vi "visuallyInspectPositionListResults2.vi"() -> ()   [LabVIEW 2016]
uses:
  <vilib>/Utility/file.llb/Write Delimited Spreadsheet (DBL).vi
  <vilib>/regexp/Match Regular Expression.xnode
  <vilib>/vision/driver/NI_Vision_Acquisition_Software.lvlib
panel:
  in  "Ncaptures":i32=10
  in  "Scan height?":bool=TRUE
  in  "Stepsize [um]":dbl=200.0
  in  "Focusing test range [mm]":dbl=0.8
  in  "milliseconds to wait":u32=5000
  in  "Camera gain":dbl(slide)=5.019455252918288 scale=0.0..16.0
  in  "Nloops":i32=1
  in  "Home?":bool
  in  "Path to save collected images":path=path "C:/Users/Aerotech/Documents/Stave Assembly Records/2017-03-30/ChangeHeight/images"
  out "Finished!":bool
  out "Image #":i32=319
  out "Error report":errorcluster
  out "Most recently collected image":T1(plugin-control)
  out "XYZ Stage Current Position":T2={"X [-750, 750 mm]"=122.51800503908298, "Y [-150, 30 mm]"=-145.62509155644523, "Z [-50, 50 mm]"=10.9688762056}
  in  "Axes Speeds [mm/s]":T3={"X Speed"=10.0, "Y Speed"=10.0, "Z Speed"=10.0}
  out "Moving":bool
  in  "Camera Name":refnum<k21>="cam1" caption="IMAQdx Session"
  in  "Object Location [mm]":T4={"Go to X"=122.518, "Go to Y"=-145.6251, "Go to Z"=10.9689}
  in  "error in (no error)":errorcluster
  in  "Set of Coordinates to Process":dbl[][](array[numeric])=[[122.518, -50.0451, 9.5689], [122.518, -50.0451, 9.5689], [122.518, -50.0451, 9.5689], [122.518, -50.0451, 9.5689], [122.518, -50.0451, 9.5689], [122.518, -50.0451, 9.5689], [122.518, -50.0451, 9.5689], [122.518, -50.0451, 9.5689], [122.518, -50.0451, 9.5689], [122.518, -50.0451, 9.5689], [122.518, -50.0451, 9.768899999999999], [122.518, -50.0451, 9.768899999999999], [122.518, -50.0451, 9.768899999999999], [122.518, -50.0451, 9.768899999999999], [122.518, -50.0451, 9.768899999999999], [122.518, -50.0451, 9.768899999999999], [122.518, -50.0451, 9.768899999999999], [122.518, -50.0451, 9.768899999999999], [122.518, -50.0451, 9.768899999999999], [122.518, -50.0451, 9.768899999999999], [122.518, -50.0451, 9.9689], [122.518, -50.0451, 9.9689], [122.518, -50.0451, 9.9689], [122.518, -50.0451, 9.9689], [122.518, -50.0451, 9.9689], [122.518, -50.0451, 9.9689], [122.518, -50.0451, 9.9689], [122.518, -50.0451, 9.9689], [122.518, -50.0451, 9.9689], [122.518, -50.0451, 9.9689], [122.518, -50.0451, 10.168899999999999], [122.518, -50.0451, 10.168899999999999], [122.518, -50.0451, 10.168899999999999], [122.518, -50.0451, 10.168899999999999], [122.518, -50.0451, 10.168899999999999], [122.518, -50.0451, 10.168899999999999], [122.518, -50.0451, 10.168899999999999], [122.518, -50.0451, 10.168899999999999], [122.518, -50.0451, 10.168899999999999], [122.518, -50.0451, 10.168899999999999], [122.518, -50.0451, 10.3689], [122.518, -50.0451, 10.3689], [122.518, -50.0451, 10.3689], [122.518, -50.0451, 10.3689], [122.518, -50.0451, 10.3689], [122.518, -50.0451, 10.3689], [122.518, -50.0451, 10.3689], [122.518, -50.0451, 10.3689], [122.518, -50.0451, 10.3689], [122.518, -50.0451, 10.3689], [122.518, -50.0451, 10.5689], [122.518, -50.0451, 10.5689], [122.518, -50.0451, 10.5689], [122.518, -50.0451, 10.5689], [122.518, -50.0451, 10.5689], [122.518, -50.0451, 10.5689], [122.518, -50.0451, 10.5689], [122.518, -50.0451, 10.5689], [122.518, -50.0451, 10.5689], [122.518, -50.0451, 10.5689], [122.518, -50.0451, 10.768899999999999], [122.518, -50.0451, 10.768899999999999], [122.518, -50.0451, 10.768899999999999], [122.518, -50.0451, 10.768899999999999], [122.518, -50.0451, 10.768899999999999], [122.518, -50.0451, 10.768899999999999], [122.518, -50.0451, 10.768899999999999], [122.518, -50.0451, 10.768899999999999], [122.518, -50.0451, 10.768899999999999], [122.518, -50.0451, 10.768899999999999], [122.518, -50.0451, 10.9689], [122.518, -50.0451, 10.9689], [122.518, -50.0451, 10.9689], [122.518, -50.0451, 10.9689], [122.518, -50.0451, 10.9689], [122.518, -50.0451, 10.9689], [122.518, -50.0451, 10.9689], [122.518, -50.0451, 10.9689], [122.518, -50.0451, 10.9689], [122.518, -50.0451, 10.9689], [218.098, -50.0451, 9.5689], [218.098, -50.0451, 9.5689], [218.098, -50.0451, 9.5689], [218.098, -50.0451, 9.5689], [218.098, -50.0451, 9.5689], [218.098, -50.0451, 9.5689], [218.098, -50.0451, 9.5689], [218.098, -50.0451, 9.5689], [218.098, -50.0451, 9.5689], [218.098, -50.0451, 9.5689], [218.098, -50.0451, 9.768899999999999], [218.098, -50.0451, 9.768899999999999], [218.098, -50.0451, 9.768899999999999], [218.098, -50.0451, 9.768899999999999], [218.098, -50.0451, 9.768899999999999], [218.098, -50.0451, 9.768899999999999], [218.098, -50.0451, 9.768899999999999], [218.098, -50.0451, 9.768899999999999], [218.098, -50.0451, 9.768899999999999], [218.098, -50.0451, 9.768899999999999], [218.098, -50.0451, 9.9689], [218.098, -50.0451, 9.9689], [218.098, -50.0451, 9.9689], [218.098, -50.0451, 9.9689], [218.098, -50.0451, 9.9689], [218.098, -50.0451, 9.9689], [218.098, -50.0451, 9.9689], [218.098, -50.0451, 9.9689], [218.098, -50.0451, 9.9689], [218.098, -50.0451, 9.9689], [218.098, -50.0451, 10.168899999999999], [218.098, -50.0451, 10.168899999999999], [218.098, -50.0451, 10.168899999999999], [218.098, -50.0451, 10.168899999999999], [218.098, -50.0451, 10.168899999999999], [218.098, -50.0451, 10.168899999999999], [218.098, -50.0451, 10.168899999999999], [218.098, -50.0451, 10.168899999999999], [218.098, -50.0451, 10.168899999999999], [218.098, -50.0451, 10.168899999999999], [218.098, -50.0451, 10.3689], [218.098, -50.0451, 10.3689], [218.098, -50.0451, 10.3689], [218.098, -50.0451, 10.3689], [218.098, -50.0451, 10.3689], [218.098, -50.0451, 10.3689], [218.098, -50.0451, 10.3689], [218.098, -50.0451, 10.3689], [218.098, -50.0451, 10.3689], [218.098, -50.0451, 10.3689], [218.098, -50.0451, 10.5689], [218.098, -50.0451, 10.5689], [218.098, -50.0451, 10.5689], [218.098, -50.0451, 10.5689], [218.098, -50.0451, 10.5689], [218.098, -50.0451, 10.5689], [218.098, -50.0451, 10.5689], [218.098, -50.0451, 10.5689], [218.098, -50.0451, 10.5689], [218.098, -50.0451, 10.5689], [218.098, -50.0451, 10.768899999999999], [218.098, -50.0451, 10.768899999999999], [218.098, -50.0451, 10.768899999999999], [218.098, -50.0451, 10.768899999999999], [218.098, -50.0451, 10.768899999999999], [218.098, -50.0451, 10.768899999999999], [218.098, -50.0451, 10.768899999999999], [218.098, -50.0451, 10.768899999999999], [218.098, -50.0451, 10.768899999999999], [218.098, -50.0451, 10.768899999999999], [218.098, -50.0451, 10.9689], [218.098, -50.0451, 10.9689], [218.098, -50.0451, 10.9689], [218.098, -50.0451, 10.9689], [218.098, -50.0451, 10.9689], [218.098, -50.0451, 10.9689], [218.098, -50.0451, 10.9689], [218.098, -50.0451, 10.9689], [218.098, -50.0451, 10.9689], [218.098, -50.0451, 10.9689], [218.098, -145.6251, 9.5689], [218.098, -145.6251, 9.5689], [218.098, -145.6251, 9.5689], [218.098, -145.6251, 9.5689], [218.098, -145.6251, 9.5689], [218.098, -145.6251, 9.5689], [218.098, -145.6251, 9.5689], [218.098, -145.6251, 9.5689], [218.098, -145.6251, 9.5689], [218.098, -145.6251, 9.5689], [218.098, -145.6251, 9.768899999999999], [218.098, -145.6251, 9.768899999999999], [218.098, -145.6251, 9.768899999999999], [218.098, -145.6251, 9.768899999999999], [218.098, -145.6251, 9.768899999999999], [218.098, -145.6251, 9.768899999999999], [218.098, -145.6251, 9.768899999999999], [218.098, -145.6251, 9.768899999999999], [218.098, -145.6251, 9.768899999999999], [218.098, -145.6251, 9.768899999999999], [218.098, -145.6251, 9.9689], [218.098, -145.6251, 9.9689], [218.098, -145.6251, 9.9689], [218.098, -145.6251, 9.9689], [218.098, -145.6251, 9.9689], [218.098, -145.6251, 9.9689], [218.098, -145.6251, 9.9689], [218.098, -145.6251, 9.9689], [218.098, -145.6251, 9.9689], [218.098, -145.6251, 9.9689], [218.098, -145.6251, 10.168899999999999], [218.098, -145.6251, 10.168899999999999], [218.098, -145.6251, 10.168899999999999], [218.098, -145.6251, 10.168899999999999], [218.098, -145.6251, 10.168899999999999], [218.098, -145.6251, 10.168899999999999], [218.098, -145.6251, 10.168899999999999], [218.098, -145.6251, 10.168899999999999], [218.098, -145.6251, 10.168899999999999], [218.098, -145.6251, 10.168899999999999], [218.098, -145.6251, 10.3689], [218.098, -145.6251, 10.3689], [218.098, -145.6251, 10.3689], [218.098, -145.6251, 10.3689], [218.098, -145.6251, 10.3689], [218.098, -145.6251, 10.3689], [218.098, -145.6251, 10.3689], [218.098, -145.6251, 10.3689], [218.098, -145.6251, 10.3689], [218.098, -145.6251, 10.3689], [218.098, -145.6251, 10.5689], [218.098, -145.6251, 10.5689], [218.098, -145.6251, 10.5689], [218.098, -145.6251, 10.5689], [218.098, -145.6251, 10.5689], [218.098, -145.6251, 10.5689], [218.098, -145.6251, 10.5689], [218.098, -145.6251, 10.5689], [218.098, -145.6251, 10.5689], [218.098, -145.6251, 10.5689], [218.098, -145.6251, 10.768899999999999], [218.098, -145.6251, 10.768899999999999], [218.098, -145.6251, 10.768899999999999], [218.098, -145.6251, 10.768899999999999], [218.098, -145.6251, 10.768899999999999], [218.098, -145.6251, 10.768899999999999], [218.098, -145.6251, 10.768899999999999], [218.098, -145.6251, 10.768899999999999], [218.098, -145.6251, 10.768899999999999], [218.098, -145.6251, 10.768899999999999], [218.098, -145.6251, 10.9689], [218.098, -145.6251, 10.9689], [218.098, -145.6251, 10.9689], [218.098, -145.6251, 10.9689], [218.098, -145.6251, 10.9689], [218.098, -145.6251, 10.9689], [218.098, -145.6251, 10.9689], [218.098, -145.6251, 10.9689], [218.098, -145.6251, 10.9689], [218.098, -145.6251, 10.9689], [122.518, -145.6251, 9.5689], [122.518, -145.6251, 9.5689], [122.518, -145.6251, 9.5689], [122.518, -145.6251, 9.5689], [122.518, -145.6251, 9.5689], [122.518, -145.6251, 9.5689], [122.518, -145.6251, 9.5689], [122.518, -145.6251, 9.5689], [122.518, -145.6251, 9.5689], [122.518, -145.6251, 9.5689], [122.518, -145.6251, 9.768899999999999], [122.518, -145.6251, 9.768899999999999], [122.518, -145.6251, 9.768899999999999], [122.518, -145.6251, 9.768899999999999], [122.518, -145.6251, 9.768899999999999], [122.518, -145.6251, 9.768899999999999], [122.518, -145.6251, 9.768899999999999], [122.518, -145.6251, 9.768899999999999], [122.518, -145.6251, 9.768899999999999], [122.518, -145.6251, 9.768899999999999], [122.518, -145.6251, 9.9689], [122.518, -145.6251, 9.9689], [122.518, -145.6251, 9.9689], [122.518, -145.6251, 9.9689], [122.518, -145.6251, 9.9689], [122.518, -145.6251, 9.9689], [122.518, -145.6251, 9.9689], [122.518, -145.6251, 9.9689], [122.518, -145.6251, 9.9689], [122.518, -145.6251, 9.9689], [122.518, -145.6251, 10.168899999999999], [122.518, -145.6251, 10.168899999999999], [122.518, -145.6251, 10.168899999999999], [122.518, -145.6251, 10.168899999999999], [122.518, -145.6251, 10.168899999999999], [122.518, -145.6251, 10.168899999999999], [122.518, -145.6251, 10.168899999999999], [122.518, -145.6251, 10.168899999999999], [122.518, -145.6251, 10.168899999999999], [122.518, -145.6251, 10.168899999999999], [122.518, -145.6251, 10.3689], [122.518, -145.6251, 10.3689], [122.518, -145.6251, 10.3689], [122.518, -145.6251, 10.3689], [122.518, -145.6251, 10.3689], [122.518, -145.6251, 10.3689], [122.518, -145.6251, 10.3689], [122.518, -145.6251, 10.3689], [122.518, -145.6251, 10.3689], [122.518, -145.6251, 10.3689], [122.518, -145.6251, 10.5689], [122.518, -145.6251, 10.5689], [122.518, -145.6251, 10.5689], [122.518, -145.6251, 10.5689], [122.518, -145.6251, 10.5689], [122.518, -145.6251, 10.5689], [122.518, -145.6251, 10.5689], [122.518, -145.6251, 10.5689], [122.518, -145.6251, 10.5689], [122.518, -145.6251, 10.5689], [122.518, -145.6251, 10.768899999999999], [122.518, -145.6251, 10.768899999999999], [122.518, -145.6251, 10.768899999999999], [122.518, -145.6251, 10.768899999999999], [122.518, -145.6251, 10.768899999999999], [122.518, -145.6251, 10.768899999999999], [122.518, -145.6251, 10.768899999999999], [122.518, -145.6251, 10.768899999999999], [122.518, -145.6251, 10.768899999999999], [122.518, -145.6251, 10.768899999999999], [122.518, -145.6251, 10.9689], [122.518, -145.6251, 10.9689], [122.518, -145.6251, 10.9689], [122.518, -145.6251, 10.9689], [122.518, -145.6251, 10.9689], [122.518, -145.6251, 10.9689], [122.518, -145.6251, 10.9689], [122.518, -145.6251, 10.9689], [122.518, -145.6251, 10.9689], [122.518, -145.6251, 10.9689]]
  in  "File delimiter":string=","
  in  "List of Interesting Locations":path=path "C:/Users/Aerotech/Documents/Stave Assembly Records/2017-03-30/ChangeHeight/corners.csv"
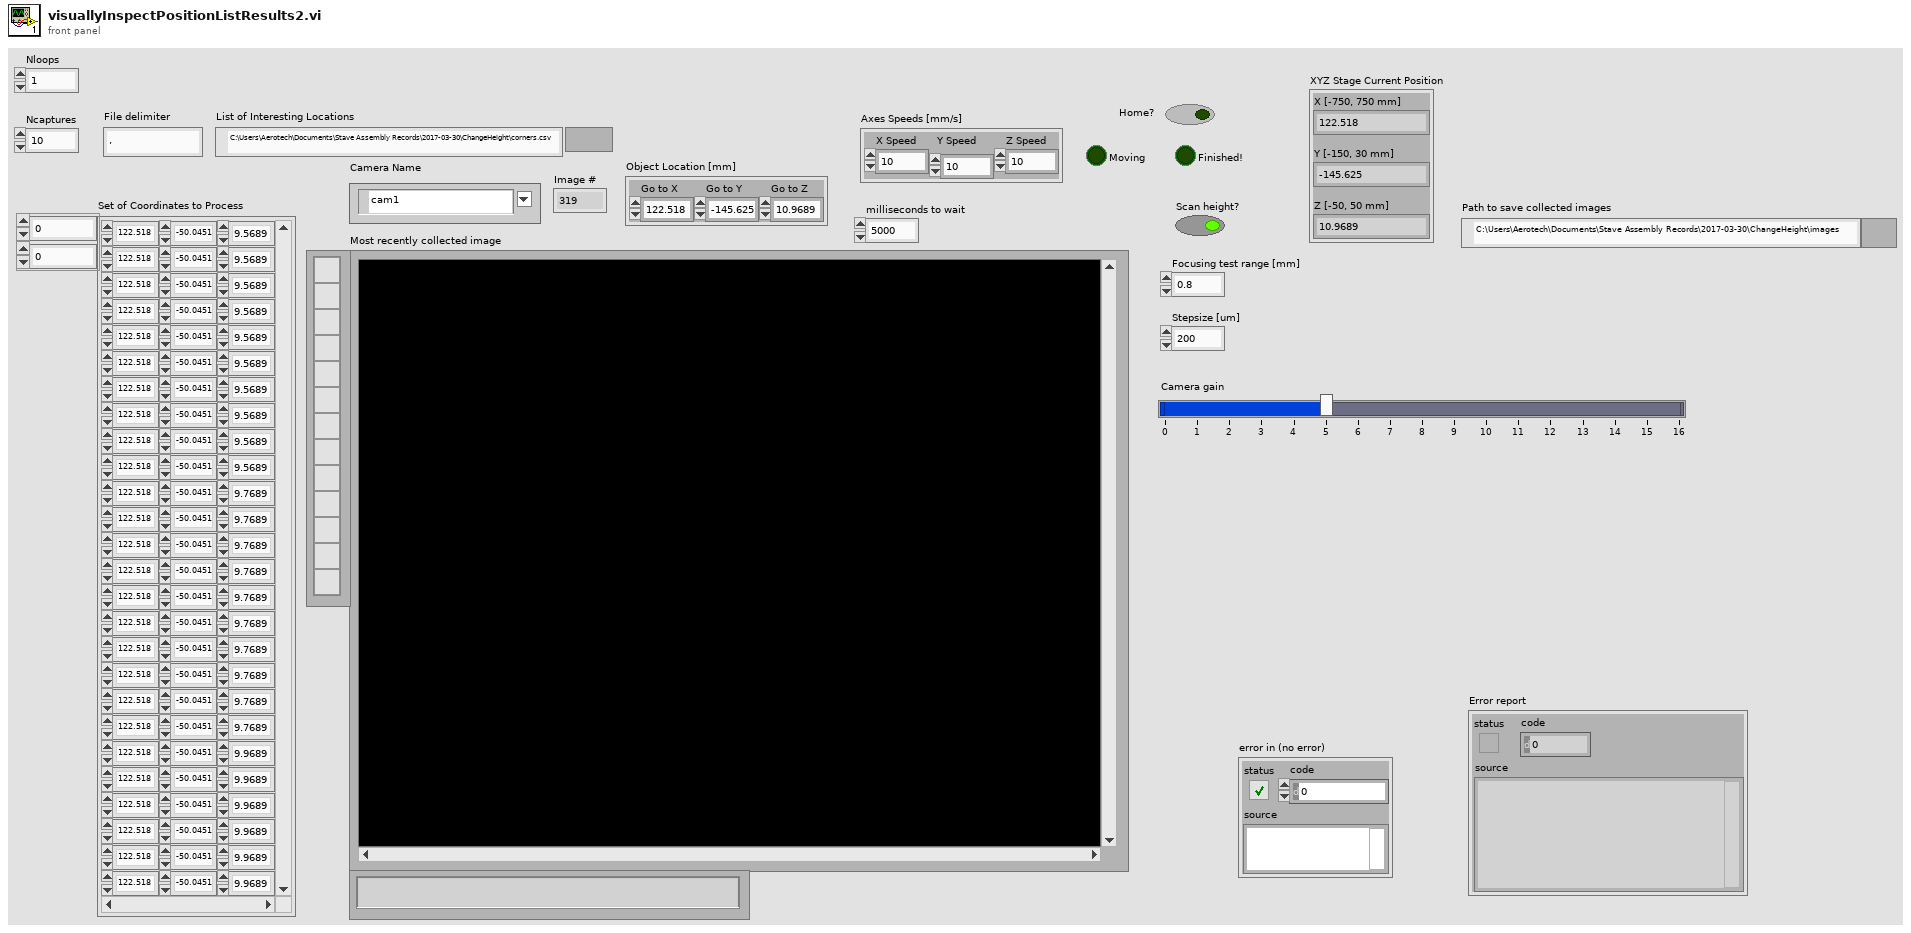
[diagram p1: front panel]
types:
  T1 = typedef "IMAQ Image.ctl" = refnum<image>
  T2 = cluster{"X [-750, 750 mm]":dbl, "Y [-150, 30 mm]":dbl, "Z [-50, 50 mm]":dbl}
  T3 = cluster{"X Speed":dbl, "Y Speed":dbl, "Z Speed":dbl}
  T4 = cluster{"Go to X":dbl, "Go to Y":dbl, "Go to Z":dbl}
  T5 = cluster{"Loaded array[0]":dbl, "Loaded array[1]":dbl, "Loaded array[2]":dbl, "Loaded array[3]":dbl, "Loaded array[4]":dbl, "Loaded array[5]":dbl, "Loaded array[6]":dbl, "Loaded array[7]":dbl, "Loaded array[8]":dbl}
  T6 = typedef "IMAQdx.ctl" = refnum<k21>
  T7 = cluster{"Set of Coordinates to Process[0]":dbl, "Set of Coordinates to Process[1]":dbl, "Set of Coordinates to Process[2]":dbl}
  T8 = typedef "Image Type" = u32
  T9 = cluster{"Final X":dbl, "Final Y":dbl, "Final Z":dbl}
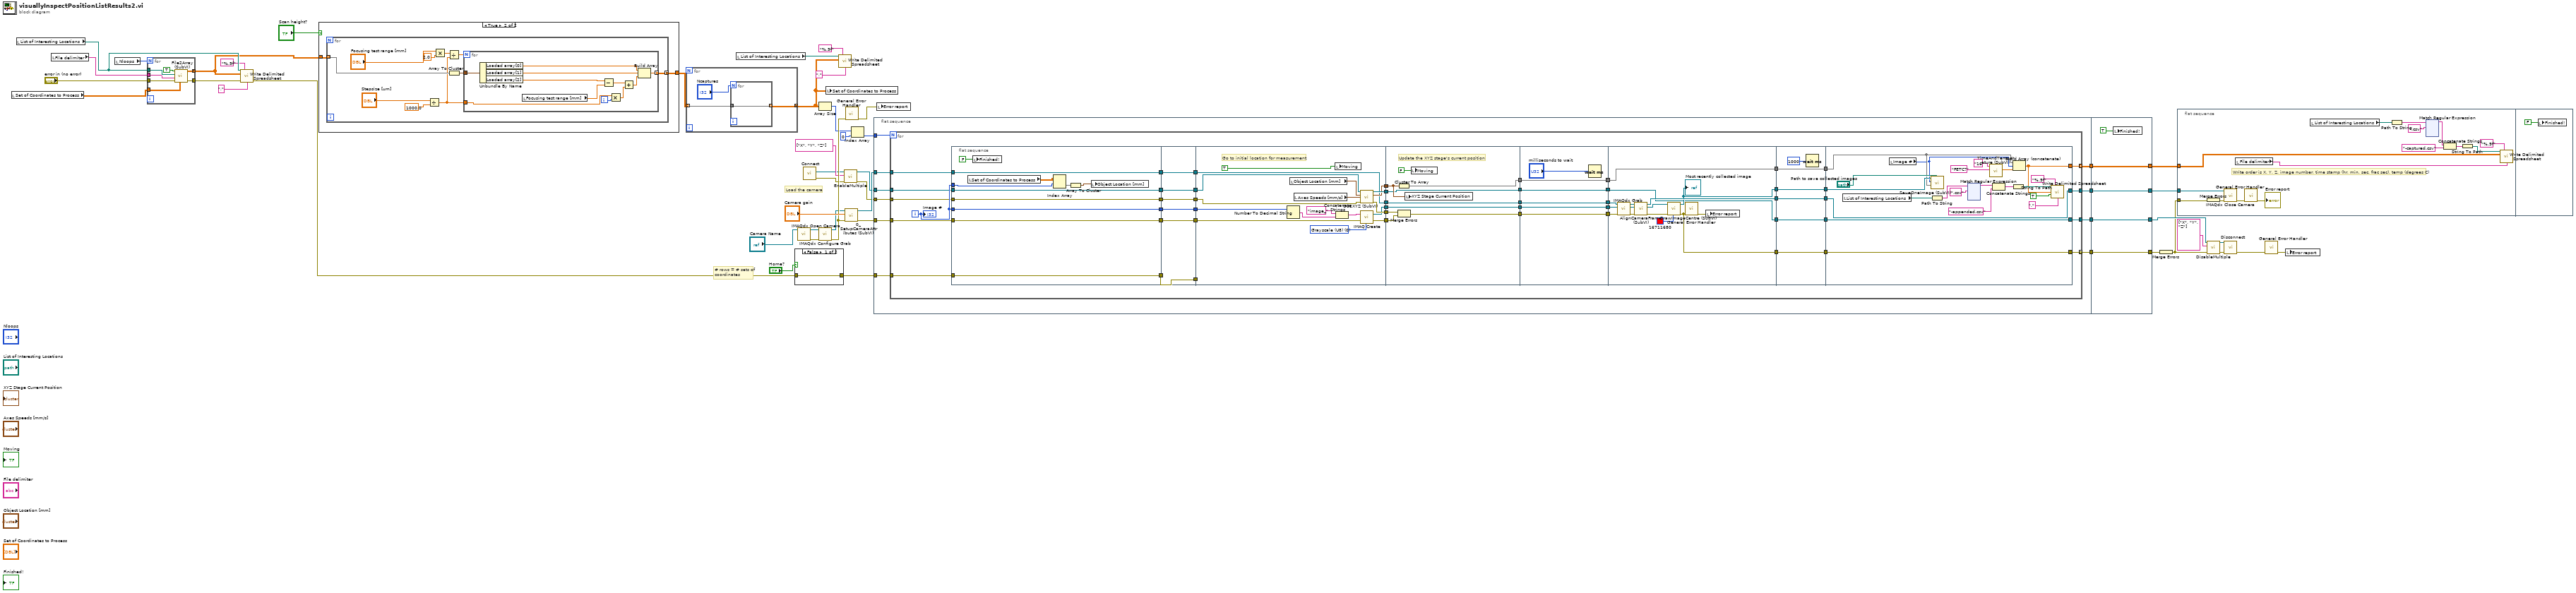
[diagram p0: block diagram]
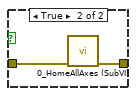
[diagram p3: hidden frame]
diagram:
  # "# rows = # sets of\ncoordinates"
  # "Load the camera"
  n1 = local read "Set of Coordinates to Process"() -> (w35:dbl[][])
  n2 = local read "List of Interesting Locations"() -> (w34:path)
  n3 = local read "File delimiter"() -> (w37:string)
  n4 = local read "Nloops"() -> (w4:i32)
  n5 = for {
    N: w4 -> [_]
    tunnel: w34 -> [w53]
    tunnel: w37 -> [w52]
    tunnel: w35 -> [w50]
    tunnel: [w56] -> w11 mode=concatenating
    tunnel: "error in (no error)" -> [w51]
    tunnel: [w55] -> w2
    n6 = call "File2Array (SubVI).vi"("Array for Processing"=w50, "error in (no error) in"=w51, "File delimiter"=w52, "Source array file"=w53, "Load array from file?"=TRUE) -> ("error in (no error) out"=w55:errorcluster, "Loaded array"=w56:dbl[][])  [unwired: 5 in]
  }
  n7 = call-poly <vilib>:"Write Delimited Spreadsheet.vi"("file path (dialog if empty)"=w34, "format (%.3f)"="%.9f", "2D data"=w11, "error in (no error)"=w2, "delimiter (\\t)"="," ("delimiter (\\t)")) -> ("error out"=w42:errorcluster)  [unwired: 9 in, 1 out]
  n8 = case shown="True" "Scan height?" {
    tunnel: w11 -> [w57 w59]
    tunnel: [w57 w58] -> w10
    frame False {
    }
    frame True {
      n9 = for {
        tunnel: w59 -> [w65] mode=indexing
        tunnel: [w63] -> w58 mode=concatenating
        n10 = Divide(x="Stepsize [um]", y=1000.0) -> (x/y=w60:dbl)
        n11 = Multiply(x="Focusing test range [mm]", y=2.0) -> (x*y=w67:dbl)
        n12 = Divide(x=w67, y=w60) -> (x/y=w68:dbl)
        n13 = Array To Cluster(array=w65) -> (cluster=w64:T5)
        n14 = for {
          N: w68 -> [_]
          tunnel: w64 -> [w80]
          tunnel: [w77] -> w63 mode=indexing
          tunnel: w60 -> [w75]
          i -> [w76]
          n15 = Unbundle By Name(w80) -> ("Loaded array[0]"=w79:dbl, "Loaded array[1]"=w78:dbl, "Loaded array[2]"=w74:dbl)
          n16 = local read "Focusing test range [mm]"() -> (w73:dbl)
          n17 = Subtract(x=w74, y=w73) -> (x-y=w72:dbl)
          n18 = Multiply(x=w75, y=w76) -> (x*y=w71:dbl)
          n19 = Add(x=w72, y=w71) -> (x+y=w70:dbl)
          n20 = Build Array(w79, w78, w70) -> (w77:dbl[])
        }
      }
    }
  }
  n21 = for {
    tunnel: w10 -> [w82] mode=indexing
    tunnel: [w81] -> w5 mode=concatenating
    n22 = for {
      N: "Ncaptures" -> [_]
      tunnel: w82 -> [w84]
      tunnel: [w84] -> w81 mode=indexing
    }
  }
  n23 = local read "List of Interesting Locations"() -> (w8:path)
  n24 = case shown="False" "Home?" {
    tunnel: w42 -> [w85 w87]
    tunnel: [w85 w86] -> w41
    frame False {
    }
    frame True {
      n25 = call "0_HomeAllAxes (SubVI).vi"("error in (no error)"=w87) -> ("error out"=w86:errorcluster)  [unwired: 7 in, 3 out]
    }
  }
  n26 = call <vilib>:"IMAQdx Open Camera.vi"("Session In"="Camera Name") -> ("error out"=w46:errorcluster, "Session Out"=w47:T6)  [unwired: 2 in, 7 out]
  n27 = call "Connect.vi"() -> ("error out"=w23:errorcluster, "controller"=w22:refnum<k24>)  [unwired: 10 in]
  n28 = Array Size(array=w5) -> (size(s)=w9:i32[])
  n29 = call <vilib>:"IMAQdx Configure Grab.vi"("error in"=w46, "Session In"=w47) -> ("error out"=w29:errorcluster, "Session Out"=w28:T6)  [unwired: 8 out]
  n30 = local write "Set of Coordinates to Process"(w5) -> ()
  n31 = call-poly <vilib>:"Write Delimited Spreadsheet.vi"("file path (dialog if empty)"=w8, "format (%.3f)"="%.9f", "2D data"=w5, "delimiter (\\t)"="," ("delimiter (\\t)")) -> ()  [unwired: 10 in, 2 out]
  n32 = call "EnableMultiple.vi"("error in (no error)"=w23, "axis names"=string[] ["X", "Y", "Z"], "controller in"=w22) -> ("error out"=w20:errorcluster, "controller out"=w21:refnum<k24>)  [unwired: 7 in]
  n33 = call "0_SetupCameraAttributes (SubVI).vi"("error in (no error)"=w29, "Gain"="Camera gain", "Camera session in"=w28) -> ("error out"=w26:errorcluster, "Camera session out"=w27:T6)  [unwired: 7 in]
  n34 = call <vilib>:"General Error Handler.vi"("error in (no error)"=w29) -> ("error out"=w39:errorcluster)  [unwired: 2 in, 12 out]
  n35 = Index Array(array=w9, index=0) -> (element=w48:i32)
  n36 = flat-sequence {
    tunnel: w48 -> [w97]
    tunnel: w27 -> [w96]
    tunnel: w41 -> [w94]
    tunnel: w26 -> [w92]
    tunnel: [w95] -> w33
    tunnel: [w88] -> w32
    tunnel: [w93] -> w31
    tunnel: w21 -> [w91]
    tunnel: w20 -> [w90]
    tunnel: [w89] -> w19
    tunnel: [w353] -> w40
    tunnel: [w354] -> w43
    tunnel: [w355] -> w44
    tunnel: w33 -> [w355]
    tunnel: w32 -> [w354]
    tunnel: w31 -> [w353]
    tunnel: [w351] -> w17
    tunnel: w19 -> [w351]
    frame #0 {
      n37 = for {
        N: w97 -> [_]
        tunnel: w96 -> [w135]
        tunnel: w94 -> [w134]
        tunnel: w92 -> [w133]
        tunnel: [w129] -> w95
        tunnel: [w128] -> w93 mode=indexing
        tunnel: w91 -> [w117]
        tunnel: w90 -> [w116]
        tunnel: [w111] -> w89
        tunnel: [w110] -> w88 mode=indexing
        i -> [w142]
        n38 = flat-sequence {
          tunnel: w142 -> [w153]
          tunnel: w142 -> [w152]
          tunnel: [w152] -> w109
          tunnel: [w151] -> w107
          tunnel: w135 -> [w151]
          tunnel: [w150] -> w105
          tunnel: w134 -> [w150]
          tunnel: [w149] -> w103
          tunnel: w133 -> [w149]
          tunnel: [w147] -> w101
          tunnel: w117 -> [w147]
          tunnel: w116 -> [w146]
          tunnel: [w146] -> w99
          tunnel: w109 -> [w162]
          tunnel: [w162] -> w108
          tunnel: w107 -> [w161]
          tunnel: [w161] -> w106
          tunnel: w105 -> [w160]
          tunnel: [w160] -> w104
          tunnel: w103 -> [w159]
          tunnel: [w159] -> w102
          tunnel: w101 -> [w158]
          tunnel: [w158] -> w100
          tunnel: w99 -> [w157]
          tunnel: [w157] -> w98
          tunnel: [w175] -> w145
          tunnel: [w174] -> w144
          tunnel: [w173] -> w143
          tunnel: w108 -> [w168]
          tunnel: [w170] -> w139
          tunnel: [w169] -> w136
          tunnel: w106 -> [w169]
          tunnel: w104 -> [_]
          tunnel: w102 -> [w166]
          tunnel: [w165] -> w130
          tunnel: w100 -> [w164]
          tunnel: w98 -> [w163]
          tunnel: w145 -> [w180]
          tunnel: w144 -> [w183]
          tunnel: w143 -> [w181]
          tunnel: [w187] -> w140
          tunnel: w139 -> [w187]
          tunnel: [w186] -> w137
          tunnel: w136 -> [w186]
          tunnel: [w184] -> w131
          tunnel: w130 -> [w185]
          tunnel: [w182] -> w127
          tunnel: [w180] -> w115
          tunnel: [w193] -> w141
          tunnel: w140 -> [w193]
          tunnel: [w192] -> w138
          tunnel: w137 -> [w192]
          tunnel: [w191] -> w132
          tunnel: w131 -> [w191]
          tunnel: w127 -> [w190]
          tunnel: [w190] -> w126
          tunnel: w115 -> [w189]
          tunnel: [w189] -> w114
          tunnel: w141 -> [w209]
          tunnel: w138 -> [w208]
          tunnel: w132 -> [w206]
          tunnel: w126 -> [w204]
          tunnel: [w199] -> w125
          tunnel: [w198] -> w124
          tunnel: [w204] -> w123
          tunnel: [w197] -> w119
          tunnel: w114 -> [w195]
          tunnel: [w195] -> w112
          tunnel: w125 -> [w215]
          tunnel: w124 -> [w214]
          tunnel: w123 -> [w213]
          tunnel: [w215] -> w122
          tunnel: [w214] -> w121
          tunnel: [w213] -> w120
          tunnel: w119 -> [w211]
          tunnel: [w211] -> w118
          tunnel: [w210] -> w113
          tunnel: w112 -> [w210]
          tunnel: [w235] -> w128
          tunnel: [w236] -> w129
          tunnel: w122 -> [w236]
          tunnel: w121 -> [w235]
          tunnel: w120 -> [w229]
          tunnel: w118 -> [w234]
          tunnel: [w232] -> w111
          tunnel: w113 -> [w232]
          tunnel: [w218] -> w110
          frame #0 {
            n39 = local read "Set of Coordinates to Process"() -> (w154:dbl[][])
            n40 = local write "Finished!"(FALSE ("Finished!")) -> ()
            n41 = Index Array(array=w154, index (row)=w153) -> (element=w155:dbl[])  [unwired: 1 in]
            n42 = Array To Cluster(array=w155) -> (cluster=w156:T7)
            n43 = local write "Object Location [mm]"(w156) -> ()
          }
          frame #1 {
          }
          frame #2 {
            w179 = T8 0 items=["Grayscale (U8)", "Grayscale (I16)", "Grayscale (SGL)", "Complex (CSG)", "RGB (U32)", "HSL (U32)", "RGB (U64)", "Grayscale (U16)"] ("Image Type")
            # "Go to initial location for measurement"
            n44 = Number To Decimal String(number=w168) -> (decimal integer string=w167:string)  [unwired: 1 in]
            n45 = local read "Object Location [mm]"() -> (w176:T4)
            n46 = local read "Axes Speeds [mm/s]"() -> (w177:T3)
            n47 = local write "Moving"(TRUE ("Moving")) -> ()
            n48 = Concatenate Strings("image_" ("Image Name"), w167) -> (w171:string)
            n49 = call "Go2XYZ (SubVI).vi"(".NET Refnum in"=w164, "Go to Coordinates"=w176, "Axis Speeds"=w177, "error in (no error)"=w163) -> (".NET Refnum out"=w175:refnum<k24>, "Final Position"=w174:T9, "error out"=w173:errorcluster)  [unwired: 7 in, 2 out]
            n50 = call "IMAQ Create"("Image Name"=w171, "Image Type"=w179, "error in (no error)"=w166) -> ("New Image"=w170:T1, "error out"=w165:errorcluster)  [unwired: 1 in, 1 out]
          }
          frame #3 {
            # "Update the XYZ stage's current position"
            n51 = Cluster To Array(cluster=w183) -> (array=w182:dbl[])
            n52 = Merge Errors(w181, w185) -> (w184:errorcluster)
            n53 = local write "XYZ Stage Current Position"(w183) -> ()
            n54 = local write "Moving"(FALSE ("Moving")) -> ()
          }
          frame #4 {
            n55 = Wait (ms)(milliseconds to wait="milliseconds to wait") -> ()  [unwired: 1 out]
          }
          frame #5 {
            n56 = call <vilib>:"IMAQdx Grab.vi"("error in"=w206, "Image In"=w209, "Session In"=w208) -> ("error out"=w205:errorcluster, "Image Out"=w207:T1, "Session Out"=w200:T6)  [unwired: 1 in, 5 out]
            n57 = call "AlignCameraFrame (SubVI).vi"("error in (no error)"=w205, "Image Src"=w207, "Camera session in"=w200) -> ("error out"=w202:errorcluster, "Image Dst Out"=w203:T1, "Camera session out"=w199:T6)  [unwired: 6 in]
            n58 = call "DrawImageCentre (SubVI).vi"("Axis colour"=u32 16711680, "error in (no error)"=w202, "Refnum in"=w203) -> ("error out"=w198:errorcluster, "Refnum out"=w197:T1)  [unwired: 7 in]
            "Most recently collected image" <- w197
            n59 = call <vilib>:"General Error Handler.vi"("error in (no error)"=w198) -> ("error out"=w196:errorcluster)  [unwired: 2 in, 12 out]
            n60 = local write "Error report"(w196) -> ()
          }
          frame #6 {
            n61 = Wait (ms)(milliseconds to wait=u32 1000) -> ()  [unwired: 1 out]
          }
          frame #7 {
            n62 = local read "List of Interesting Locations"() -> (w226:path)
            n63 = local read "Image #"() -> (w227:i32)
            n64 = Path To String(path=w226) -> (string=w225:string)
            n65 = call "SaveOneImage (SubVI).vi"("Save images path"="Path to save collected images", "XYZ stage coordinates of image"=w229, "Image Number"=w227, "Image"=w234) -> ()  [unwired: 7 in, 1 out]
            n66 = xnode "Match Regular Expression"("input string"=w225, "regular expression"=".csv") -> ("before match"=w222:string)  [unwired: 4 in, 4 out]
            n67 = call "TimeAndTemperature (SubVI).vi"("Command"="FETC?", "GPIB Address: Temperature"="16") -> ("double( Time, Temp )"=w228:dbl[])  [unwired: 6 in, 3 out]
            n68 = Concatenate Strings(w222, "-appended.csv" ("name or relative path")) -> (w221:string)
            n69 = String To Path(string=w221) -> (path=w220:path)
            n70 = Build Array (concatenate)(w229, w227, w228) -> (w218:dbl[])
            n71 = call-poly <vilib>:"Write Delimited Spreadsheet.vi"("file path (dialog if empty)"=w220, "format (%.3f)"="%.9f", "1D data"=w218, "append to file? (new file:F)"=TRUE, "delimiter (\\t)"="," ("delimiter (\\t)")) -> ()  [unwired: 9 in, 2 out]
          }
        }
        "Image #" <- w142
      }
    }
    frame #1 {
      n72 = local write "Finished!"(TRUE ("Finished!")) -> ()
    }
  }
  n73 = local write "Error report"(w39) -> ()
  n74 = Merge Errors(w40) -> (w15:errorcluster)
  n75 = flat-sequence {
    tunnel: w15 -> [w360]
    tunnel: w44 -> [w359]
    tunnel: w43 -> [w358]
    frame #0 {
      # "Write order is X, Y, Z, image number, time stamp (hr, min, sec, frac sec), temp (degrees C)"
      n76 = Merge Errors(w360) -> (w361:errorcluster)
      n77 = call <vilib>:"IMAQdx Close Camera.vi"("error in"=w361, "Session In"=w359) -> ("error out"=w357:errorcluster)  [unwired: 9 out]
      n78 = local read "File delimiter"() -> (w370:string)
      n79 = call <vilib>:"General Error Handler.vi"("error in (no error)"=w357) -> ("error out"=→"Error report":errorcluster)  [unwired: 2 in, 12 out]
      n80 = local read "List of Interesting Locations"() -> (w363:path)
      n81 = Path To String(path=w363) -> (string=w364:string)
      n82 = xnode "Match Regular Expression"("input string"=w364, "regular expression"=".csv") -> ("before match"=w367:string)  [unwired: 4 in, 4 out]
      n83 = Concatenate Strings(w367, "-captured.csv" ("name or relative path")) -> (w368:string)
      n84 = String To Path(string=w368) -> (path=w369:path)
      n85 = call-poly <vilib>:"Write Delimited Spreadsheet.vi"("file path (dialog if empty)"=w369, "format (%.3f)"="%.9f", "2D data"=w358, "delimiter (\\t)"=w370) -> ()  [unwired: 10 in, 2 out]
    }
    frame #1 {
      n86 = local write "Finished!"(FALSE ("Finished!")) -> ()
    }
  }
  n87 = call "DisableMultiple.vi"("error in (no error)"=w15, "axis names"=string[] ["X", "Y", "Z"], "controller in"=w17) -> ("error out"=w14:errorcluster, "controller out"=w16:refnum<k24>)  [unwired: 7 in]
  n88 = call "Disconnect.vi"("error in (no error)"=w14, "controller"=w16) -> ("error out"=w18:errorcluster)  [unwired: 9 in]
  n89 = call <vilib>:"General Error Handler.vi"("error in (no error)"=w18) -> ("error out"=w25:errorcluster)  [unwired: 2 in, 12 out]
  n90 = local write "Error report"(w25) -> ()
